vi "Convert to SICK array.vi"(8 "Left Regions":bool[](array[boolean]), 11 "Right Regions":bool[](array[boolean])) -> (1 "Sick array":u16[](array[numeric]))   [LabVIEW 2009]
panel:
  # "On top: Subsector data\nOn bottom: Sick sector data"
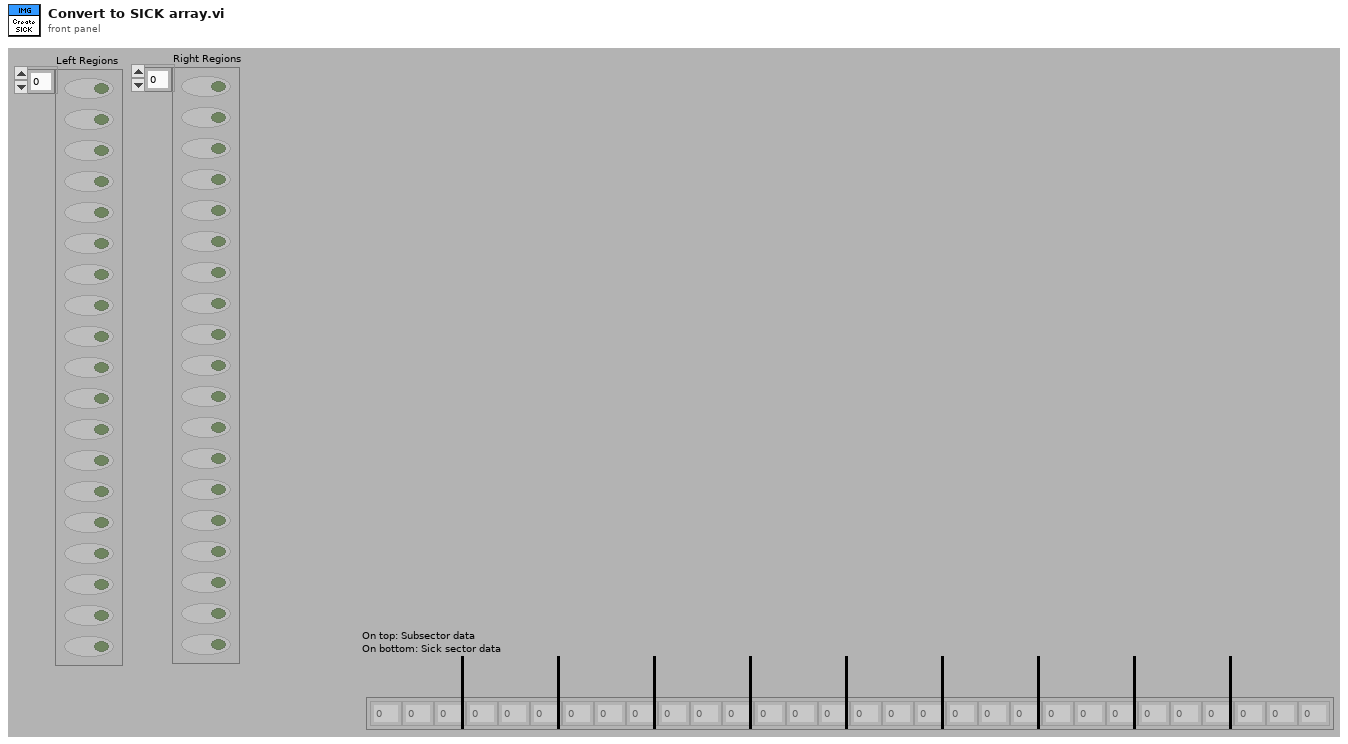
[diagram p1: front panel]
types:
  T1 = cluster{"[0]":u16, "[1]":u16, "[2]":u16, "[3]":u16, "[4]":u16}
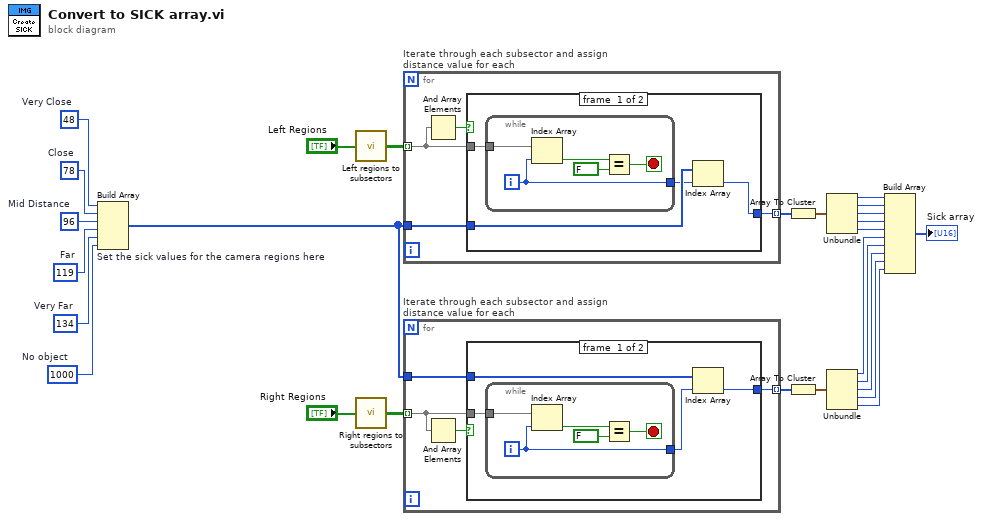
[diagram p0: block diagram]
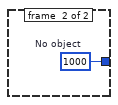
[diagram p2: hidden frame]
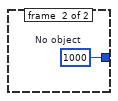
[diagram p3: hidden frame]
diagram:
  w20 = u16 1000  # No object
  w21 = u16 48  # Very Close
  w22 = u16 134  # Very Far
  w25 = u16 119  # Far
  w24 = u16 96  # Mid Distance
  w23 = u16 78  # Close
  n1 = Build Array "Set the sick values for the camera regions here"(w21, w23, w24, w25, w22, w20) -> (w18:u16[])
  n2 = call "Left regions to subsectors.vi"("Left Regions"="Left Regions") -> ("Left subsector array"=w3:bool[][])
  n3 = call "Right regions to subsectors.vi"("Right Regions"="Right Regions") -> ("Right subsector array"=w17:bool[][])
  n4 = for "Iterate through each subsector and assign distance value for each" {
    tunnel: w3 -> [w29] mode=indexing
    tunnel: w18 -> [w27]
    tunnel: [w28] -> w1 mode=indexing
    n5 = And Array Elements(Boolean array=w29) -> (logical AND=w30:bool)
    n6 = case shown="False" w30 {
      tunnel: [w31 w40] -> w28
      tunnel: w27 -> [w33 _]
      tunnel: w29 -> [w34 _]
      frame #0 {
        n7 = while {
          tunnel: w34 -> [w39]
          tunnel: [w35] -> w32
          i -> [w35]
          stop <- w36 stop-if-true
          n8 = Index Array(array=w39, index=w35) -> (element=w38:bool)
          n9 = Equal?(x=w38, y=FALSE) -> (x = y?=w36:bool)
        }
        n10 = Index Array(array=w33, index=w32) -> (element=w31:u16)
      }
      frame #1 {
        w40 = u16 1000  # No object
      }
    }
  }
  n11 = for "Iterate through each subsector and assign distance value for each" {
    tunnel: w17 -> [w42] mode=indexing
    tunnel: w18 -> [w43]
    tunnel: [w41] -> w2 mode=indexing
    n12 = And Array Elements(Boolean array=w42) -> (logical AND=w44:bool)
    n13 = case shown="False" w44 {
      tunnel: [w45 w54] -> w41
      tunnel: w43 -> [w47 _]
      tunnel: w42 -> [w48 _]
      frame #0 {
        n14 = while {
          tunnel: w48 -> [w53]
          tunnel: [w49] -> w46
          i -> [w49]
          stop <- w50 stop-if-true
          n15 = Index Array(array=w53, index=w49) -> (element=w52:bool)
          n16 = Equal?(x=w52, y=FALSE) -> (x = y?=w50:bool)
        }
        n17 = Index Array(array=w47, index=w46) -> (element=w45:u16)
      }
      frame #1 {
        w54 = u16 1000  # No object
      }
    }
  }
  n18 = Array To Cluster(array=w1) -> (cluster=w15:T1)
  n19 = Array To Cluster(array=w2) -> (cluster=w16:T1)
  n20 = Unbundle(w15) -> ("[0]"=w14:u16, "[1]"=w13:u16, "[2]"=w12:u16, "[3]"=w11:u16, "[4]"=w10:u16)
  n21 = Unbundle(w16) -> ("[0]"=w9:u16, "[1]"=w8:u16, "[2]"=w7:u16, "[3]"=w6:u16, "[4]"=w5:u16)
  n22 = Build Array(w14, w13, w12, w11, w10, w9, w8, w7, w6, w5) -> (→"Sick array":u16[])
